vi "Dual DC PS Control and Monitor.vi"() -> ()   [LabVIEW 2018]
uses:
  <vilib>/DAQmx/read.llb/DAQmx Read (Analog 1D DBL NChan 1Samp).vi
  <vilib>/DAQmx/write.llb/DAQmx Write (Analog 1D DBL NChan 1Samp).vi
  <vilib>/DAQmx/create/channels.llb/DAQmx Create Channel (AI-Voltage-Basic).vi
  <vilib>/DAQmx/create/channels.llb/DAQmx Create Channel (AI-Current-Basic).vi
  <vilib>/DAQmx/miscellaneous.llb/DAQmx Fill In Error Info.vi
  <vilib>/DAQmx/create/channels.llb/DAQmx Create Channel (AO-Voltage-Basic).vi
  <vilib>/ptbypt/NI_PtbyPt.lvlib
panel:
  out "PS 2 Amps":dbl
  out "PS 1 Amps":dbl format="%#.2f"
  in  "Scale 2":dbl=10.1
  in  "Offset 2":dbl
  out "Power Supply\nOutput VDC 2":dbl(knob) scale=0.0..36.0
  out "Numeric 4":dbl format="%.1f"
  out "Numeric 3":dbl format="%.1f"
  in  "Slide 2":dbl(slide) min=0.0 max=36.0 step=0.5 scale=0.0..36.0
  out "Control VDC 2":dbl
  in  "Output Scale 2":dbl
  in  "Output Scale":dbl
  out "Control VDC":dbl
  in  "Slide":dbl(slide) min=0.0 max=36.0 step=0.5 scale=0.0..36.0
  out "Numeric 2":dbl format="%.1f"
  out "Numeric":dbl format="%.1f"
  out "Power Supply\nOutput VDC":dbl(knob) scale=0.0..36.0
  in  "Offset":dbl
  in  "Scale":dbl=10.25
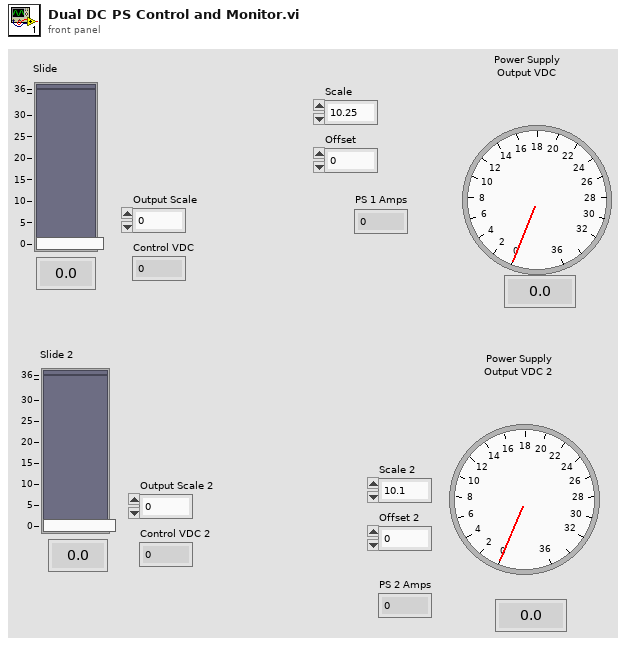
[diagram p1: front panel]
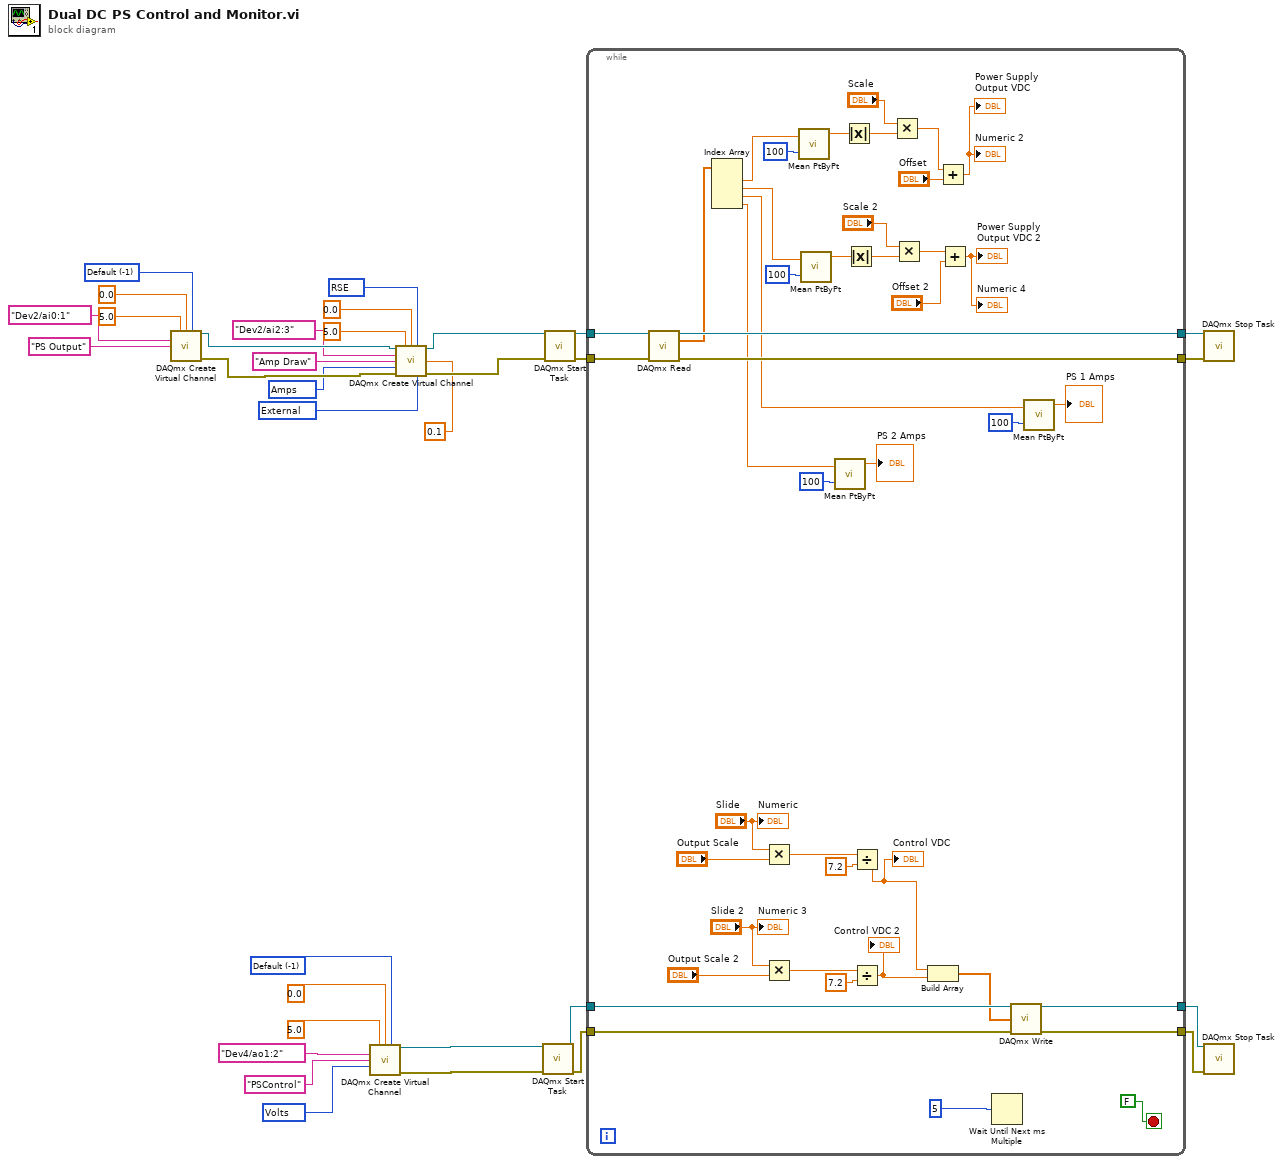
[diagram p0: block diagram]
diagram:
  w1 = 10167 items=["default"=-1, "Internal"=10200, "External"=10167] ("shunt resistor location")
  w3 = 10342 items=["Amps"=10342, "From Custom Scale"=10065] ("units")
  w6 = 10083 items=["default"=-1, "RSE"=10083, "NRSE"=10078, "Differential"=10106, "Pseudodifferential"=12529] ("input terminal configuration")
  w23 = -1 items=["Default"=-1, "RSE"=10083, "NRSE"=10078, "Differential"=10106, "Pseudodifferential"=12529] ("input terminal configuration")
  w26 = -1 items=["Default"=-1, "RSE"=10083, "Differential"=10106, "Pseudodifferential"=12529] ("output terminal configuration")
  w31 = 10348 items=["Volts"=10348, "From Custom Scale"=10065] ("units")
  n1 = call-poly <vilib>:"DAQmx Create Virtual Channel.vi"("maximum value"=5.0, "minimum value"=0.0, "input terminal configuration"=w23, "physical channels"=tag "Dev2/ai0:1", "name to assign"="PS Output") -> ("task out"=w12:refnum<k21>, "error out"=w9:errorcluster)  [unwired: 9 in]
  n2 = call-poly <vilib>:"DAQmx Create Virtual Channel.vi"("maximum value"=5.0, "minimum value"=0.0, "output terminal configuration"=w26, "physical channels"=tag "Dev4/ao1:2", "name to assign"="PSControl", "units"=w31) -> ("task out"=w32:refnum<k21>, "error out"=w33:errorcluster)  [unwired: 8 in]
  n3 = call-poly <vilib>:"DAQmx Create Virtual Channel.vi"("task in"=w12, "maximum value"=5.0, "minimum value"=0.0, "input terminal configuration"=w6, "physical channels"=tag "Dev2/ai2:3", "name to assign"="Amp Draw", "external shunt resistor value"=0.1, "units"=w3, "error in"=w9, "shunt resistor location"=w1) -> ("task out"=w11:refnum<k21>, "error out"=w10:errorcluster)  [unwired: 4 in]
  n4 = call <vilib>:"DAQmx Start Task.vi"("task/channels in"=w32, "error in"=w33) -> ("task out"=w21:refnum<k21>, "error out"=w20:errorcluster)  [unwired: 12 in]
  n5 = call <vilib>:"DAQmx Start Task.vi"("task/channels in"=w11, "error in"=w10) -> ("task out"=w17:refnum<k21>, "error out"=w16:errorcluster)  [unwired: 12 in]
  n6 = while {
    tunnel: w21 -> [w76]
    tunnel: w20 -> [w75]
    tunnel: [w74] -> w19
    tunnel: [w73] -> w18
    tunnel: w17 -> [w72]
    tunnel: w16 -> [w71]
    tunnel: [w67] -> w15
    tunnel: [w66] -> w14
    stop <- FALSE stop-if-true
    n7 = call-poly <vilib>:"DAQmx Read.vi"("task/channels in"=w72, "error in"=w71) -> ("task out"=w67:refnum<k21>, "data"=w49:dbl[], "error out"=w66:errorcluster)  [unwired: 11 in]
    n8 = Index Array(array=w49) -> (element #1=w41:dbl, element #2=w40:dbl, element #3=w39:dbl, element #4=w36:dbl)  [unwired: 4 in]
    n9 = Multiply(x="Slide", y="Output Scale") -> (x*y=w59:dbl)
    n10 = Multiply(x="Slide 2", y="Output Scale 2") -> (x*y=w55:dbl)
    n11 = call <vilib>:"Mean PtByPt.vi"("x"=w41, "sample length"=100) -> ("mean"=w63:dbl)  [unwired: 2 in, 1 out]
    n12 = call <vilib>:"Mean PtByPt.vi"("x"=w40, "sample length"=100) -> ("mean"=w47:dbl)  [unwired: 2 in, 1 out]
    n13 = call <vilib>:"Mean PtByPt.vi"("x"=w36, "sample length"=100) -> ("mean"=→"PS 2 Amps":dbl)  [unwired: 2 in, 1 out]
    n14 = Absolute Value(x=w63) -> (abs(x)=w57:dbl)
    n15 = Absolute Value(x=w47) -> (abs(x)=w48:dbl)
    n16 = Divide(x=w59, y=7.2) -> (x/y=w51:dbl)
    "Control VDC" <- w51
    n17 = Divide(x=w55, y=7.2) -> (x/y=w50:dbl)
    "Control VDC 2" <- w50
    n18 = Multiply(x="Scale", y=w57) -> (x*y=w68:dbl)
    n19 = Multiply(x="Scale 2", y=w48) -> (x*y=w44:dbl)
    n20 = Build Array(w51, w50) -> (w52:dbl[])
    n21 = Add(x=w68, y="Offset") -> (x+y=→"Power Supply\nOutput VDC" →"Numeric 2":dbl)
    n22 = Add(x=w44, y="Offset 2") -> (x+y=→"Power Supply\nOutput VDC 2" →"Numeric 4":dbl)
    n23 = Wait Until Next ms Multiple(millisecond multiple=u32 5) -> ()  [unwired: 1 out]
    n24 = call-poly <vilib>:"DAQmx Write.vi"("task/channels in"=w76, "data"=w52, "error in"=w75) -> ("task out"=w74:refnum<k21>, "error out"=w73:errorcluster)  [unwired: 10 in, 1 out]
    n25 = call <vilib>:"Mean PtByPt.vi"("x"=w39, "sample length"=100) -> ("mean"=→"PS 1 Amps":dbl)  [unwired: 2 in, 1 out]
    "Numeric" <- "Slide"
    "Numeric 3" <- "Slide 2"
  }
  n26 = call <vilib>:"DAQmx Stop Task.vi"("task/channels in"=w15, "error in"=w14) -> ()  [unwired: 12 in, 2 out]
  n27 = call <vilib>:"DAQmx Stop Task.vi"("task/channels in"=w19, "error in"=w18) -> ()  [unwired: 12 in, 2 out]
